vi "FrameUnpack.vi"(8 "error in":errorcluster caption="错误输入", 9 "FilePath":string, 10 "RegisterIn":T2, 11 "FramePack":string="\u0002\u0001þ\u0000\u00002F0´Xk0UM¨:n+|Ý#include <stdio.h>\n#include <stdlib.h>\n#include <string.h>\n\n#include <sys/types.h>\n#include <sys/stat.h>\n#include <unistd.h>\n#include <fcntl.h>\n\n#include \"common.h\"\n#include \"xmodem_file_transport.h\"\n#include \"upload_dload.h\"\n\n\n#define MIN_UPLOAD_FIRST_DATA_LEN  (PACKAGE_DATA_LEN_128 - 4 - 16)\n\n\n/*====================== globle datas define =============================*/\ntypedef struct{\n\tunsigned char package_head;\n\tunsigned char package_num;\n\tunsigned char package_num_flag;\n\tint upload_data_len;\n}last_upload_fileinfo;\n\ntypedef struct{\n\tint file_fd;\n\tint file_len;\n\tunsigned char file_md5[FILE_MD5_NUMS];\n}upload_file_info;\n\nupload_file_info m_upload_file_info = {0};\nlast_upload_fileinfo m_last_upload_fileinfo = {0};\nxmodem_timer m_upload_timer = {0};\nstatic int m_send_file_len = -1; \n\n/*===================  upload file functions begin  ======================*/\ninline void judge_last_package_num()\n{\n\tif(ACK_ACK == m_upload_timer.ack_flag){\n\t\tif(0xFF == m_last_upload_fileinfo.package_num){\n\t\t\u0001\u0000\u0000\u0000­\u0000\n\u0000\u0000") -> (0 "error out":errorcluster caption="错误输出", 1 "RegisterOut":T1, 2 "当前接收包序号":u32, 3 "CRC？":bool)   [LabVIEW 2013]
uses:
  RegisterPara.ctl
panel:
  out "x = y?":bool
  out "长度":i32
  out "MD5_1":string
  out "MD":string
  out "MD5":string
  out "CRCStr":string
  out "子字符串":string
  out "CRC":string
  out "FileText":string
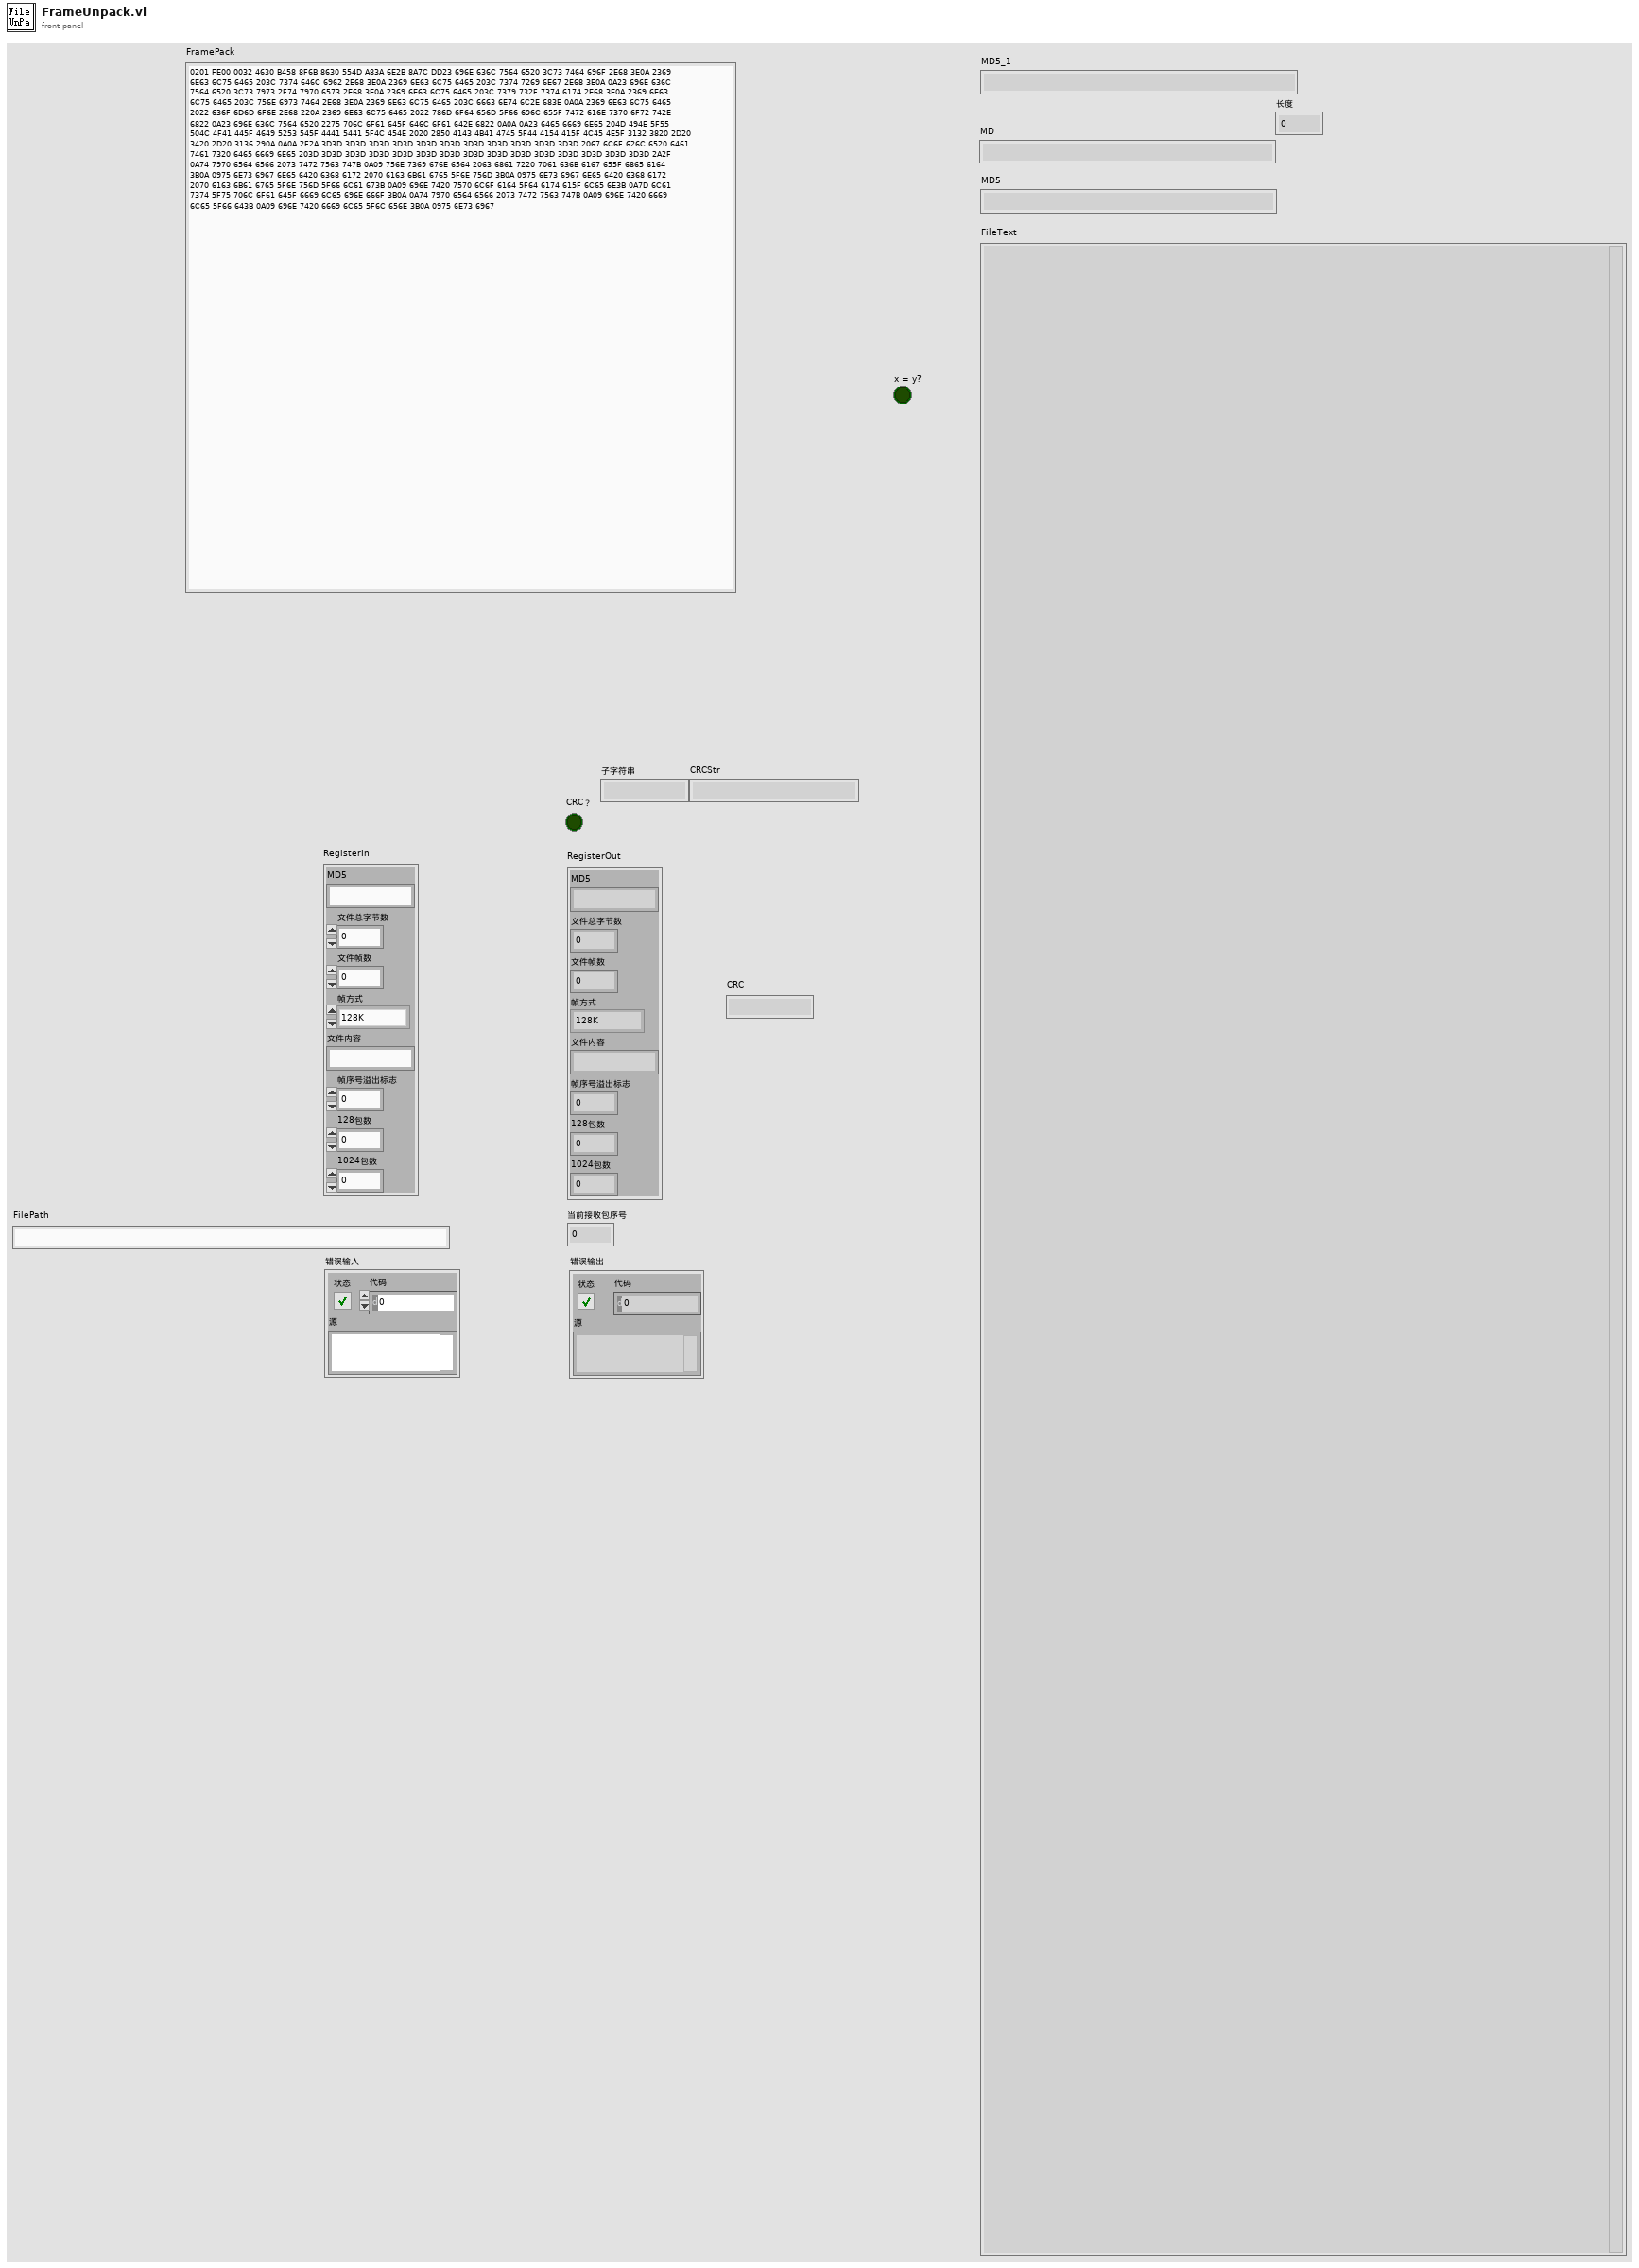
[diagram p1: front panel]
types:
  T1 = typedef "RegisterPara.ctl" = cluster{"MD5":string, "文件总字节数":u32, "文件帧数":u32, "帧方式":enum16{"128K", "1024K-128K"}, "文件内容":string, "帧序号溢出标志":u32, "128包数":u32, "1024包数":u32}
  T2 = cluster{"MD5":string, "文件总字节数":u32, "文件帧数":u32, "帧方式":enum16{"128K", "1024K-128K"}, "文件内容":string, "帧序号溢出标志":u32, "128包数":u32, "1024包数":u32}
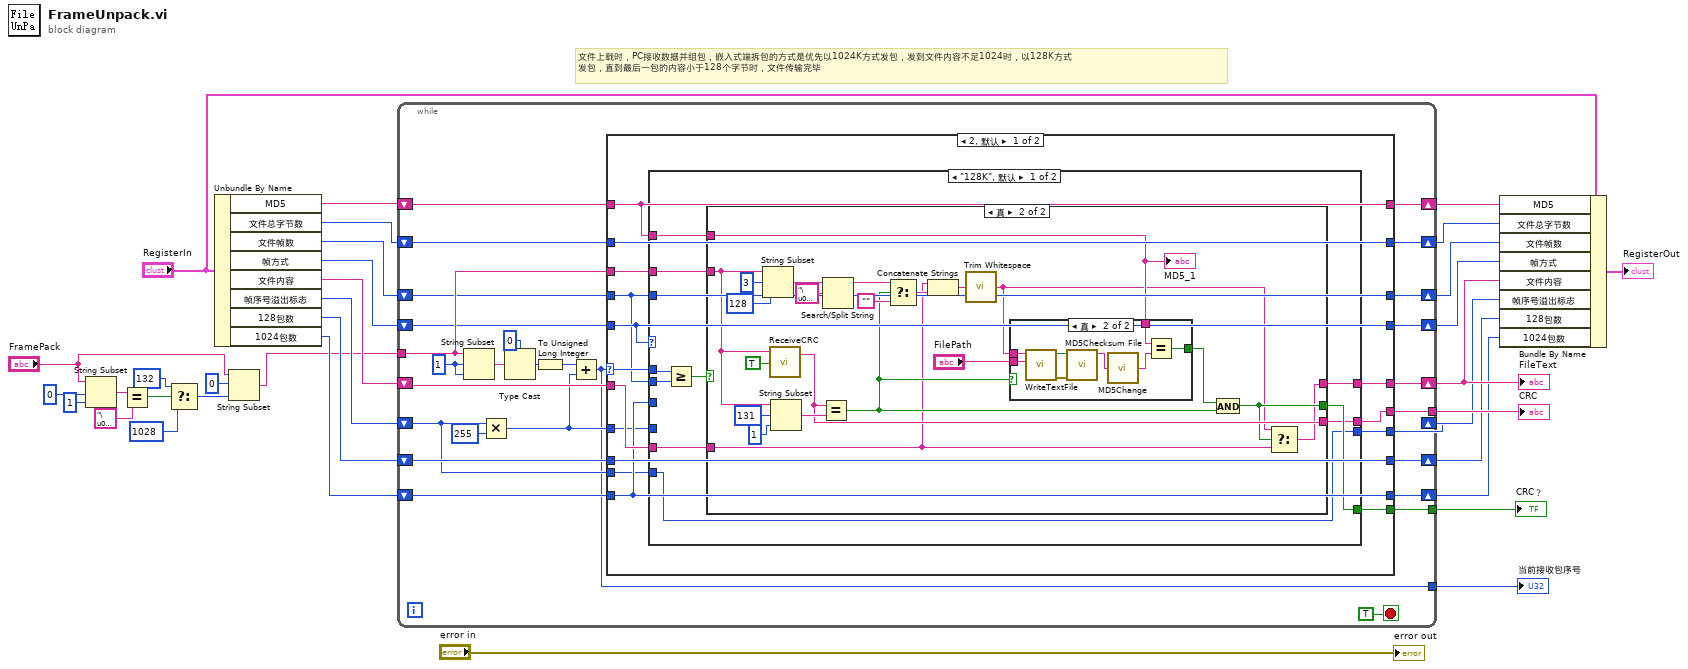
[diagram p0: block diagram]
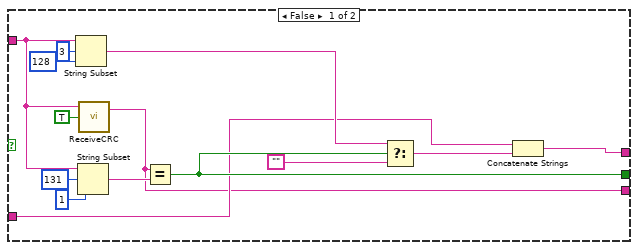
[diagram p2: hidden frame]
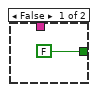
[diagram p3: hidden frame]
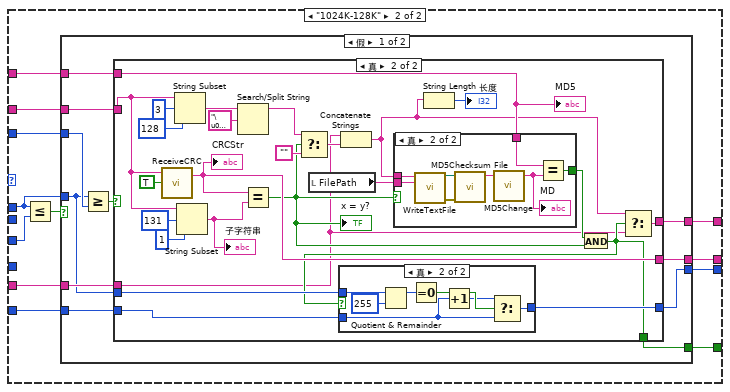
[diagram p4: hidden frame]
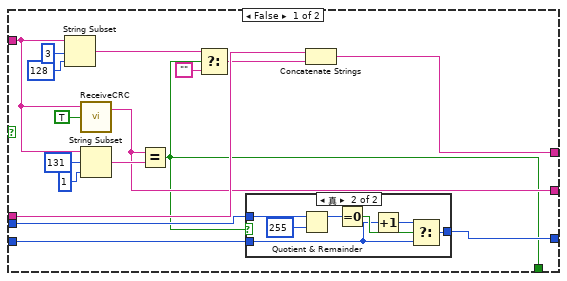
[diagram p5: hidden frame]
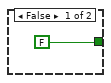
[diagram p8: hidden frame]
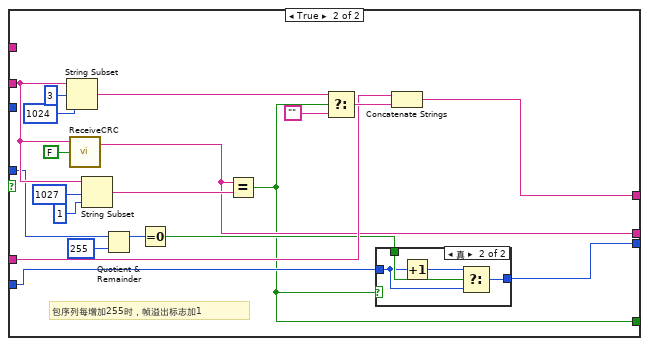
[diagram p9: hidden frame]
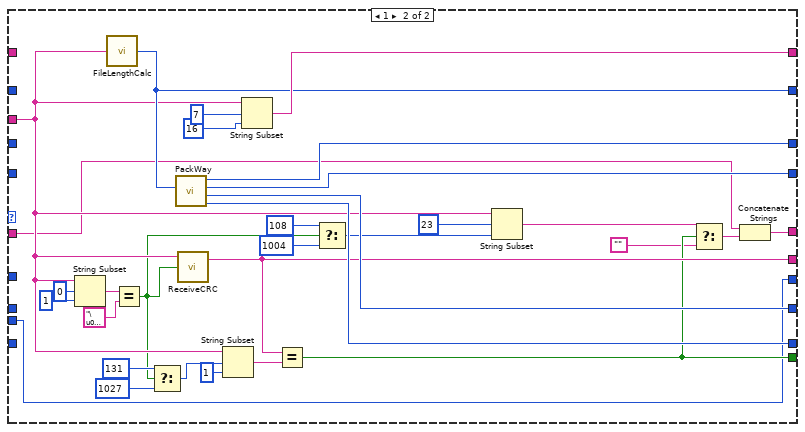
[diagram p11: hidden frame]
diagram:
  # "文件上载时，PC接收数据并组包，嵌入式端拆包的方式是优先以1024K方式发包，发到文件内容不足1024时，以128K方式\n发包，直到最后一包的内容小于128个字节时，文件传输完毕"
  n1 = String Subset(string="FramePack", offset (0)=0 ("长度（剩余）"), length (rest)=1 ("长度（剩余）")) -> (substring=w10:string)
  n2 = Equal?(x=w10, y="\u0001") -> (x = y?=w7:bool)
  n3 = Select(t=132, s=w7, f=1028) -> (s? t:f=w2:i32)
  n4 = Unbundle By Name("RegisterIn") -> ("MD5"=w30:string, "文件总字节数"=w29:u32, "文件帧数"=w28:u32, "帧方式"=w27:enum16{"128K", "1024K-128K"}, "文件内容"=w26:string, "帧序号溢出标志"=w25:u32, "128包数"=w24:u32, "1024包数"=w23:u32)
  n5 = String Subset(string="FramePack", offset (0)=0 ("长度（剩余）"), length (rest)=w2) -> (substring=w8:string)
  n6 = while {
    tunnel: w8 -> [w60]
    shift-right: [w53] -> w20
    shift-left: w30 -> [w52]
    shift-right: [w51] -> w19
    shift-left: w29 -> [w50]
    shift-right: [w49] -> w18
    shift-left: w28 -> [w48]
    shift-right: [w47] -> w17
    shift-left: w27 -> [w46]
    shift-right: [w45] -> w14
    shift-left: w24 -> [w44]
    shift-right: [w43] -> w13
    shift-left: w23 -> [w42]
    tunnel: [w41] -> w32
    tunnel: [w40] -> w31
    shift-right: [w39] -> w16
    shift-left: w26 -> [w38]
    shift-right: [w35] -> w15
    shift-left: w25 -> [w36]
    tunnel: [w34] -> w12
    stop <- TRUE stop-if-true
    w61 = 1 ("偏移量(0)")
    n7 = String Subset(string=w60, offset (0)=w61, length (rest)=w61) -> (substring=w57:string)
    n8 = Multiply(x=w36, y=u32 255 ("偏移量(0)")) -> (x*y=w37:u32)
    n9 = Type Cast(type=u8 0, x=w57) -> (*(type *) &x=w56:u8)
    n10 = To Unsigned Long Integer(number=w56) -> (unsigned 32bit integer=w55:u32)
    n11 = Add(x=w55, y=w37) -> (x+y=w34:u32)
    n12 = case shown="2, 默认" w34 {
      selector: w34 -> [w73 _]
      tunnel: w60 -> [w72 w258]
      tunnel: [w68 w275] -> w53
      tunnel: w52 -> [w68 _]
      tunnel: [w76 w274] -> w51
      tunnel: w50 -> [w76 _]
      tunnel: [w65 w273] -> w49
      tunnel: w48 -> [w65 _]
      tunnel: [w74 w272] -> w47
      tunnel: w46 -> [w74 _]
      tunnel: [w75 w271] -> w45
      tunnel: w44 -> [w75 _]
      tunnel: [w67 w270] -> w43
      tunnel: w42 -> [w67 _]
      tunnel: [w66 w261] -> w41
      tunnel: [w71 w254] -> w40
      tunnel: [w70 w251] -> w39
      tunnel: w38 -> [w69 w249]
      tunnel: w37 -> [w64 _]
      tunnel: w36 -> [w63 w248]
      tunnel: [w62 w248] -> w35
      frame 2, Default {
        n13 = case shown="\"128K\", 默认" w74 {
          tunnel: w73 -> [w85 w136]
          tunnel: w65 -> [w86 _]
          tunnel: w72 -> [w83 w141]
          tunnel: [w82 w138] -> w71
          tunnel: [w81 w140] -> w70
          tunnel: w69 -> [w80 w139]
          tunnel: w68 -> [w79 w132]
          tunnel: w67 -> [_ w143]
          tunnel: [w78 w137] -> w66
          tunnel: w65 -> [_ w135]
          tunnel: w64 -> [_ _]
          tunnel: w63 -> [w77 w134]
          tunnel: [w77 w133] -> w62
          frame "128K", Default {
            n14 = Greater Or Equal?(x=w85, y=w86) -> (x >= y?=w84:bool)
            n15 = case shown="真" w84 {
              tunnel: w83 -> [w99 w116]
              tunnel: [w92 w104] -> w82
              tunnel: [w89 w103] -> w81
              tunnel: w80 -> [w88 w101]
              tunnel: w79 -> [_ w106]
              tunnel: [w87 w105] -> w78
              frame False {
                n16 = String Subset(string=w99, offset (0)=3 ("偏移量(0)"), length (rest)=128 ("偏移量(0)")) -> (substring=w91:string)
                n17 = String Subset(string=w99, offset (0)=131 ("偏移量(0)"), length (rest)=1 ("偏移量(0)")) -> (substring=w96:string)
                n18 = call "ReceiveCRC.vi"("128K？"=TRUE, "StrIn"=w99) -> ("CRCStr"=w87:string)  [unwired: 1 in, 1 out]
                n19 = Equal?(x=w87, y=w96) -> (x = y?=w92:bool)
                n20 = Select(t=w91, s=w92, f="") -> (s? t:f=w93:string)
                n21 = Concatenate Strings(w88, w93) -> (w89:string)
              }
              frame True {
                n22 = String Subset(string=w116, offset (0)=3 ("偏移量(0)"), length (rest)=128 ("长度（剩余）")) -> (substring=w120:string)
                n23 = call "ReceiveCRC.vi"("128K？"=TRUE, "StrIn"=w116) -> ("CRCStr"=w105:string)  [unwired: 1 in, 1 out]
                n24 = String Subset(string=w116, offset (0)=131 ("偏移量(0)"), length (rest)=1) -> (substring=w114:string)
                n25 = Equal?(x=w105, y=w114) -> (x = y?=w108:bool)
                n26 = Search/Split String(string=w120, search string/char (-)="\u001a") -> (substring before match=w113:string)  [unwired: 1 in, 2 out]
                n27 = Select(t=w113, s=w108, f="") -> (s? t:f=w112:string)
                n28 = Concatenate Strings(w101, w112) -> (w109:string)
                n29 = call <vilib>:"Trim Whitespace.vi"("string"=w109) -> ("trimmed string"=w102:string)  [unwired: 1 in]
                n30 = case shown="真" w108 {
                  tunnel: "FilePath" -> [_ w131]
                  tunnel: w102 -> [_ w130]
                  tunnel: [FALSE w127] -> w107
                  tunnel: w106 -> [_ w126]
                  frame False {
                  }
                  frame True {
                    n31 = call "WriteTextFile.vi"("FilePath"=w131, "TextIn"=w130) -> ("error out"=w129:errorcluster, "PathOut"=w128:path)  [unwired: 8 in]
                    n32 = call <vilib>:"MD5Checksum File.vi"("error in (no error)"=w129, "Path"=w128) -> ("MD5 message-digest"=w125:string)  [unwired: 8 in, 1 out]
                    n33 = call "MD5Change.vi"("MD5_32"=w125) -> ("MD5_16"=w124:string)
                    n34 = Equal?(x=w126, y=w124) -> (x = y?=w127:bool)
                  }
                }
                n35 = And(x=w107, y=w108) -> (x .and. y?=w104:bool)
                n36 = Select(t=w102, s=w104, f=w101) -> (s? t:f=w103:string)
                "MD5_1" <- w106
              }
            }
          }
          frame "1024K-128K" {
            n37 = Less Or Equal?(x=w136, y=w143) -> (x <= y?=w142:bool)
            n38 = case shown="假" w142 {
              tunnel: w141 -> [w152 w238]
              tunnel: [w150 w231] -> w140
              tunnel: w139 -> [w151 w230]
              tunnel: [w148 w222] -> w138
              tunnel: [w149 w229] -> w137
              tunnel: w136 -> [w146 w228]
              tunnel: w135 -> [w153 _]
              tunnel: w134 -> [w145 w224]
              tunnel: [w144 w223] -> w133
              tunnel: w132 -> [w147 _]
              frame False {
                n39 = Greater Or Equal?(x=w146, y=w153) -> (x >= y?=w154:bool)
                n40 = case shown="真" w154 {
                  tunnel: w152 -> [w166 w200]
                  tunnel: w151 -> [w164 w182]
                  tunnel: [w160 w183] -> w150
                  tunnel: [w159 w196] -> w149
                  tunnel: [w155 w184] -> w148
                  tunnel: w147 -> [_ w191]
                  tunnel: w146 -> [w156 w188]
                  tunnel: w145 -> [w157 w186]
                  tunnel: [w158 w187] -> w144
                  frame False {
                    n41 = String Subset(string=w166, offset (0)=3, length (rest)=128) -> (substring=w163:string)
                    n42 = call "ReceiveCRC.vi"("128K？"=TRUE, "StrIn"=w166) -> ("CRCStr"=w159:string)  [unwired: 1 in, 1 out]
                    n43 = String Subset(string=w166, offset (0)=131, length (rest)=1) -> (substring=w165:string)
                    n44 = Equal?(x=w159, y=w165) -> (x = y?=w155:bool)
                    n45 = Select(t=w163, s=w155, f="") -> (s? t:f=w161:string)
                    n46 = case shown="真" w155 {
                      tunnel: [w172 w175] -> w158
                      tunnel: w157 -> [w172 w174]
                      tunnel: w156 -> [_ w173]
                      frame False {
                      }
                      frame True {
                        n47 = Quotient & Remainder ("商与余数")(x=w173, y=u32 255 ("长度（剩余）")) -> (x-y*floor(x/y)=w178:u32)  [unwired: 1 out]
                        n48 = Equal To 0? ("等于0？")(x=w178) -> (x = 0?=w177:bool)
                        n49 = Increment ("加1")(x=w174) -> (x+1=w176:u32)
                        n50 = Select ("选择")(t=w176, s=w177, f=w174) -> (s? t:f=w175:u32)
                      }
                    }
                    n51 = Concatenate Strings(w164, w161) -> (w160:string)
                  }
                  frame True {
                    n52 = call "ReceiveCRC.vi"("128K？"=TRUE, "StrIn"=w200) -> ("CRCStr"=w196:string)  [unwired: 1 in, 1 out]
                    "CRCStr" <- w196
                    n53 = String Subset(string=w200, offset (0)=3 ("偏移量(0)"), length (rest)=128 ("长度（剩余）")) -> (substring=w202:string)
                    n54 = String Subset(string=w200, offset (0)=131 ("长度（剩余）"), length (rest)=1 ("长度（剩余）")) -> (substring=w197:string)
                    "子字符串" <- w197
                    n55 = Search/Split String(string=w202, search string/char (-)="\u001a") -> (substring before match=w195:string)  [unwired: 1 in, 2 out]
                    n56 = Equal?(x=w196, y=w197) -> (x = y?=w189:bool)
                    "x = y?" <- w189
                    n57 = Select(t=w195, s=w189, f="") -> (s? t:f=w193:string)
                    n58 = local read "FilePath"() -> (w192:string)
                    n59 = Concatenate Strings(w182, w193) -> (w180:string)
                    n60 = case shown="真" w189 {
                      tunnel: w180 -> [_ w219]
                      tunnel: w192 -> [_ w218]
                      tunnel: w191 -> [_ w217]
                      tunnel: [FALSE w216] -> w190
                      frame False {
                      }
                      frame True {
                        n61 = call "WriteTextFile.vi"("FilePath"=w218, "TextIn"=w219) -> ("error out"=w220:errorcluster, "PathOut"=w221:path)  [unwired: 8 in]
                        n62 = call <vilib>:"MD5Checksum File.vi"("error in (no error)"=w220, "Path"=w221) -> ("MD5 message-digest"=w214:string)  [unwired: 8 in, 1 out]
                        n63 = call "MD5Change.vi"("MD5_32"=w214) -> ("MD5_16"=w215:string)
                        "MD" <- w215
                        n64 = Equal?(x=w217, y=w215) -> (x = y?=w216:bool)
                      }
                    }
                    n65 = String Length(string=w180) -> (length=→"长度":i32)
                    n66 = And(x=w190, y=w189) -> (x .and. y?=w184:bool)
                    n67 = case shown="真" w184 {
                      tunnel: w188 -> [_ w212]
                      tunnel: [w205 w211] -> w187
                      tunnel: w186 -> [w205 w206]
                      frame False {
                      }
                      frame True {
                        n68 = Quotient & Remainder ("商与余数")(x=w212, y=u32 255 ("长度（剩余）")) -> (x-y*floor(x/y)=w209:u32)  [unwired: 1 out]
                        n69 = Equal To 0? ("等于0？")(x=w209) -> (x = 0?=w208:bool)
                        n70 = Increment ("加1")(x=w206) -> (x+1=w207:u32)
                        n71 = Select ("选择")(t=w207, s=w208, f=w206) -> (s? t:f=w211:u32)
                      }
                    }
                    n72 = Select(t=w180, s=w184, f=w182) -> (s? t:f=w183:string)
                    "MD5" <- w191
                  }
                }
              }
              frame True {
                # "包序列每增加255时，帧溢出标志加1"
                n73 = String Subset(string=w238, offset (0)=3, length (rest)=1024 ("长度（剩余）")) -> (substring=w234:string)
                n74 = call "ReceiveCRC.vi"("128K？"=FALSE, "StrIn"=w238) -> ("CRCStr"=w229:string)  [unwired: 1 in, 1 out]
                n75 = String Subset(string=w238, offset (0)=1027 ("长度（剩余）"), length (rest)=1 ("长度（剩余）")) -> (substring=w235:string)
                n76 = Quotient & Remainder(x=w228, y=u32 255 ("偏移量(0)")) -> (x-y*floor(x/y)=w226:u32)  [unwired: 1 out]
                n77 = Equal To 0?(x=w226) -> (x = 0?=w225:bool)
                n78 = Equal?(x=w229, y=w235) -> (x = y?=w222:bool)
                n79 = Select(t=w234, s=w222, f="") -> (s? t:f=w232:string)
                n80 = case shown="真" w222 {
                  tunnel: w225 -> [_ w246]
                  tunnel: w224 -> [w242 w244]
                  tunnel: [w242 w243] -> w223
                  frame False {
                  }
                  frame True {
                    n81 = Increment(x=w244) -> (x+1=w245:u32)
                    n82 = Select(t=w245, s=w246, f=w244) -> (s? t:f=w243:u32)
                  }
                }
                n83 = Concatenate Strings(w230, w232) -> (w231:string)
              }
            }
          }
        }
      }
      frame 1 {
        n84 = String Subset(string=w258, offset (0)=0 ("偏移量(0)"), length (rest)=1 ("偏移量(0)")) -> (substring=w267:string)
        n85 = call "FileLengthCalc.vi"("StrIn"=w258) -> ("FileLen"=w274:u32)
        n86 = Equal?(x=w267, y="\u0001") -> (x = y?=w255:bool)
        n87 = Select(t=131 ("偏移量(0)"), s=w255, f=1027 ("偏移量(0)")) -> (s? t:f=w265:i32)
        n88 = call "PackWay.vi"("FileLen"=w274) -> ("I-1024包数"=w270:u32, "I-128包数"=w271:u32, "帧包方式"=w272:enum16{"128K", "1024K-128K"}, "帧数"=w273:u32)  [unwired: 7 in]
        n89 = call "ReceiveCRC.vi"("128K？"=w255, "StrIn"=w258) -> ("CRCStr"=w261:string)  [unwired: 1 in, 1 out]
        n90 = String Subset(string=w258, offset (0)=w265, length (rest)=1 ("长度（剩余）")) -> (substring=w262:string)
        n91 = String Subset(string=w258, offset (0)=7 ("偏移量(0)"), length (rest)=16 ("偏移量(0)")) -> (substring=w275:string)
        n92 = Equal?(x=w261, y=w262) -> (x = y?=w254:bool)
        n93 = Select(t=108 ("偏移量(0)"), s=w255, f=1004 ("偏移量(0)")) -> (s? t:f=w257:i32)
        n94 = String Subset(string=w258, offset (0)=23 ("偏移量(0)"), length (rest)=w257) -> (substring=w253:string)
        n95 = Select(t=w253, s=w254, f="") -> (s? t:f=w250:string)
        n96 = Concatenate Strings(w249, w250) -> (w251:string)
      }
    }
  }
  "FileText" <- w16
  "CRC？" <- w31
  "CRC" <- w32
  "当前接收包序号" <- w12
  n97 = Bundle By Name(cluster="RegisterIn", "MD5"=w20, "文件总字节数"=w19, "文件帧数"=w18, "帧方式"=w17, "文件内容"=w16, "帧序号溢出标志"=w15, "128包数"=w14, "1024包数"=w13) -> (→"RegisterOut":T2)
  "error out" <- "error in"
